vi "_nevstop_choosingDlg.vi"(8 "error in (no error)":errorcluster) -> (0 "error out":errorcluster, 1 "Cancelled?":bool=TRUE, 2 "QuckDrop":string, 3 "QDKS Info":T2[](array[typedef])=[{"VI Name"="Cluster AutoSizing", "VI Path"=path "C:/Program Files (x86)/National Instruments/LabVIEW 2014/resource/dialog/QuickDrop/plugins/QD_Cluster AutoSizing/Cluster AutoSizing.vi", "Default Shortcut"="U", "Assigned Shortcut"="u", "Description"="Using a float dialog to choose cluster auto-sizing type. Press `Shift` to set the contained cluster items recursively. \n\n- None\n- Size to Fit\n- Arrange Horizontally\n- Arrange Vertically\n\nDefault Shortcut - [U]"}, {"VI Name"="Align - Bottom Edges", "VI Path"=path "C:/Program Files (x86)/National Instruments/LabVIEW 2014/resource/dialog/QuickDrop/plugins/QD_Align&Distribute/Align - Bottom Edges.vi", "Default Shortcut"="v", "Assigned Shortcut"="v", "Description"="Align - Bottom Edges.vi\n"}, {"VI Name"="Align - Horizontal Centers", "VI Path"=path "C:/Program Files (x86)/National Instruments/LabVIEW 2014/resource/dialog/QuickDrop/plugins/QD_Align&Distribute/Align - Horizontal Centers.vi", "Default Shortcut"="v", "Assigned Shortcut"="", "Description"="Align - Horizontal Centers.vi"}, {"VI Name"="Align - Left Edges", "VI Path"=path "C:/Program Files (x86)/National Instruments/LabVIEW 2014/resource/dialog/QuickDrop/plugins/QD_Align&Distribute/Align - Left Edges.vi", "Default Shortcut"="v", "Assigned Shortcut"="5", "Description"="Align - Left Edges.vi"}, {"VI Name"="Align - Right Edges", "VI Path"=path "C:/Program Files (x86)/National Instruments/LabVIEW 2014/resource/dialog/QuickDrop/plugins/QD_Align&Distribute/Align - Right Edges.vi", "Default Shortcut"="v", "Assigned Shortcut"="", "Description"="Align - Right Edges.vi"}, {"VI Name"="Align - Top Edges", "VI Path"=path "C:/Program Files (x86)/National Instruments/LabVIEW 2014/resource/dialog/QuickDrop/plugins/QD_Align&Distribute/Align - Top Edges.vi", "Default Shortcut"="v", "Assigned Shortcut"="", "Description"="Align - Top Edges.vi"}, {"VI Name"="Align - Vertical Centers", "VI Path"=path "C:/Program Files (x86)/National Instruments/LabVIEW 2014/resource/dialog/QuickDrop/plugins/QD_Align&Distribute/Align - Vertical Centers.vi", "Default Shortcut"="v", "Assigned Shortcut"="", "Description"="Align - Vertical Centers.vi"}, {"VI Name"="Align and Distribute", "VI Path"=path "C:/Program Files (x86)/National Instruments/LabVIEW 2014/resource/dialog/QuickDrop/plugins/QD_Align&Distribute/Align and Distribute.vi", "Default Shortcut"="A", "Assigned Shortcut"="a", "Description"="Aligns selected items to the right, left, top or bottom or by horizontal or vertical centers by pressing r, l, t, b, h or v."}, {"VI Name"="Arrange VI Window", "VI Path"=path "C:/Program Files (x86)/National Instruments/LabVIEW 2014/resource/dialog/QuickDrop/plugins/QD_Arrange VI Window/Arrange VI Window.vi", "Default Shortcut"="F", "Assigned Shortcut"="f", "Description"="When used on the front panel:\n-Arranges controls and indicators to be consistent with the connector pane arrangement. \n-Resizes and moves the front panel to a consistent top left location on the primary monitor.\n\nWhen used on the block diagram:\n-Scrolls the block diagram to a reasonable location relative to the top-most and/or left-most diagram object.\n-Resizes and moves the block diagram to a consistent top left location on the primary monitor.\n\nDefault Shortcut - [F]"}, {"VI Name"="Build Array of References", "VI Path"=path "C:/Program Files (x86)/National Instruments/LabVIEW 2014/resource/dialog/QuickDrop/plugins/QD_Build Array of References/Build Array of References_NEVSTOP.vi", "Default Shortcut"="B", "Assigned Shortcut"="b", "Description"="### Build Array of Reference/Build Cluster of Reference\n\nCreate references with 'Build Array'/'buddle' together.\n\nDefault Shortcut - [B]"}, {"VI Name"="Build Cluster Of Reference", "VI Path"=path "C:/Program Files (x86)/National Instruments/LabVIEW 2014/resource/dialog/QuickDrop/plugins/QD_Build Cluster of References/Build Cluster Of Reference.vi", "Default Shortcut"="$", "Assigned Shortcut"="2", "Description"="Write a 1-2 sentence description of the functionality of your plugin here.  Replace the \"$\" below with the character you wish to assign as the default shortcut for this plugin.  Do not add any text after the 'Default Shortcut' line below.\n\nDefault Shortcut - [$]"}, {"VI Name"="Clone Control", "VI Path"=path "C:/Program Files (x86)/National Instruments/LabVIEW 2014/resource/dialog/QuickDrop/plugins/QD_Clone Control/Clone Control.vi", "Default Shortcut"="", "Assigned Shortcut"="", "Description"="Clones the selected Control(s) or Indicator(s) on the Front Panel but changes Controls to Indicators and vice versa.  In addition, if found on the Connector Pane, will attempt to place the newly created control on the opposite (left / right) side of the Connector Pane.\nNote: This script only supports the following patterns: 4x2x2x4, 5x3x3x5, 6x4x4x6, and 8x6x6x8.\n\nDefault Shortcut - [A]"}, {"VI Name"="Cluster AutoSizing - Arrange Horizontally", "VI Path"=path "C:/Program Files (x86)/National Instruments/LabVIEW 2014/resource/dialog/QuickDrop/plugins/QD_Cluster AutoSizing/Cluster AutoSizing - Arrange Horizontally.vi", "Default Shortcut"="v", "Assigned Shortcut"="", "Description"="Cluster AutoSizing - Arrange Horizontally.vi"}, {"VI Name"="Cluster AutoSizing - Arrange Veritcally", "VI Path"=path "C:/Program Files (x86)/National Instruments/LabVIEW 2014/resource/dialog/QuickDrop/plugins/QD_Cluster AutoSizing/Cluster AutoSizing - Arrange Veritcally.vi", "Default Shortcut"="v", "Assigned Shortcut"="", "Description"="Cluster AutoSizing - Arrange Veritcally.vi"}, {"VI Name"="Cluster AutoSizing - None", "VI Path"=path "C:/Program Files (x86)/National Instruments/LabVIEW 2014/resource/dialog/QuickDrop/plugins/QD_Cluster AutoSizing/Cluster AutoSizing - None.vi", "Default Shortcut"="v", "Assigned Shortcut"="", "Description"="Cluster AutoSizing - None.vi"}, {"VI Name"="Cluster AutoSizing - Size to Fit", "VI Path"=path "C:/Program Files (x86)/National Instruments/LabVIEW 2014/resource/dialog/QuickDrop/plugins/QD_Cluster AutoSizing/Cluster AutoSizing - Size to Fit.vi", "Default Shortcut"="v", "Assigned Shortcut"="", "Description"="Cluster AutoSizing - Size to Fit.vi"}, {"VI Name"="ColourUpStructures", "VI Path"=path "C:/Program Files (x86)/National Instruments/LabVIEW 2014/resource/dialog/QuickDrop/plugins/QD_ColourUpStructures/ColourUpStructures.vi", "Default Shortcut"="s", "Assigned Shortcut"="s", "Description"="Colour Up Structures."}, {"VI Name"="Copy Boolean Caption to BooleanText", "VI Path"=path "C:/Program Files (x86)/National Instruments/LabVIEW 2014/resource/dialog/QuickDrop/plugins/QD_Controls Operation/Copy Boolean Caption to BooleanText.vi", "Default Shortcut"="d", "Assigned Shortcut"="", "Description"="Copy selected boolean's caption to boolean text. If the booleans have no caption, label Text will be used instead."}, {"VI Name"="Create a Place VI Contents", "VI Path"=path "C:/Program Files (x86)/National Instruments/LabVIEW 2014/resource/dialog/QuickDrop/plugins/QD_Create a Place VI Contents/Create a Place VI Contents.vi", "Default Shortcut"="G", "Assigned Shortcut"="g", "Description"="(Note: The following shortcut was originally posted by Jarrod S. on the NI Forums here.  I decided to give his shortcut a more permanent home in the Quick Drop Enthusiasts group.)\n \nThis Quick Drop Keyboard Shortcut allows you to create a Place VI Contents VI (formerly called a \"Merge VI\") of your diagram selection and automatically create a user.lib palette entry for it, so that you can easily drop that selection of code in the future.  Follow these steps to use this shortcut:\n \nSave the attached VI in your <LabVIEW>\\resource\\dialog\\QuickDrop\\plugins folder.  No LabVIEW restart is required.\nSelect something on your diagram that you wish to make into a Place VI Contents VI.\nPress Ctrl-Space-Ctrl-Shift-G.\nSpecify a name for this Place VI Contents VI.\nCreate an icon\n \nNow you have a Place VI Contents VI that contains this diagram selection that you can use from your palettes (or Quick Drop).  Note that in step (3) above, if you had pressed Ctrl-Space-Ctrl-G instead, the palettes would not be refreshed automatically, and you would have to restart LabVIEW in order to use the new Place VI Contents VI.\n \nNote:  All Place VI Contents VIs that are created with this shortcut are stored in <LabVIEW Data>\\QuickDrop Templates.  The actual .mnu files that provide the palette entries are stored in <LabVIEW>\\user.lib\\QuickDrop Templates Palette.mnu.\n\n\nDefault Shortcut - [G]"}, {"VI Name"="Disable Controls", "VI Path"=path "C:/Program Files (x86)/National Instruments/LabVIEW 2014/resource/dialog/QuickDrop/plugins/QD_Controls Operation/Disable Controls.vi", "Default Shortcut"="l", "Assigned Shortcut"="l", "Description"="Disable Controls"}, {"VI Name"="Disable&Grayout Controls", "VI Path"=path "C:/Program Files (x86)/National Instruments/LabVIEW 2014/resource/dialog/QuickDrop/plugins/QD_Controls Operation/Disable&Grayout Controls.vi", "Default Shortcut"="l", "Assigned Shortcut"="", "Description"="Disable and grayout Controls"}, {"VI Name"="Distribute - Bottom Edges", "VI Path"=path "C:/Program Files (x86)/National Instruments/LabVIEW 2014/resource/dialog/QuickDrop/plugins/QD_Align&Distribute/Distribute - Bottom Edges.vi", "Default Shortcut"="v", "Assigned Shortcut"="", "Description"="Distribute - Bottom Edges.vi"}, {"VI Name"="Distribute - Horizontal Centers", "VI Path"=path "C:/Program Files (x86)/National Instruments/LabVIEW 2014/resource/dialog/QuickDrop/plugins/QD_Align&Distribute/Distribute - Horizontal Centers.vi", "Default Shortcut"="v", "Assigned Shortcut"="", "Description"="Distribute - Horizontal Centers.vi"}, {"VI Name"="Distribute - Horizontal Compress", "VI Path"=path "C:/Program Files (x86)/National Instruments/LabVIEW 2014/resource/dialog/QuickDrop/plugins/QD_Align&Distribute/Distribute - Horizontal Compress.vi", "Default Shortcut"="v", "Assigned Shortcut"="", "Description"="Distribute - Horizontal Compress.vi"}, {"VI Name"="Distribute - Horizontal Gap", "VI Path"=path "C:/Program Files (x86)/National Instruments/LabVIEW 2014/resource/dialog/QuickDrop/plugins/QD_Align&Distribute/Distribute - Horizontal Gap.vi", "Default Shortcut"="v", "Assigned Shortcut"="", "Description"="Distribute - Horizontal Gap.vi"}, {"VI Name"="Distribute - Left Edges", "VI Path"=path "C:/Program Files (x86)/National Instruments/LabVIEW 2014/resource/dialog/QuickDrop/plugins/QD_Align&Distribute/Distribute - Left Edges.vi", "Default Shortcut"="v", "Assigned Shortcut"="", "Description"="Distribute - Left Edges.vi"}, {"VI Name"="Distribute - Right Edges", "VI Path"=path "C:/Program Files (x86)/National Instruments/LabVIEW 2014/resource/dialog/QuickDrop/plugins/QD_Align&Distribute/Distribute - Right Edges.vi", "Default Shortcut"="v", "Assigned Shortcut"="", "Description"="Distribute - Right Edges.vi"}, {"VI Name"="Distribute - Top Edges", "VI Path"=path "C:/Program Files (x86)/National Instruments/LabVIEW 2014/resource/dialog/QuickDrop/plugins/QD_Align&Distribute/Distribute - Top Edges.vi", "Default Shortcut"="v", "Assigned Shortcut"="", "Description"="Distribute - Top Edges.vi"}, {"VI Name"="Distribute - Vertical Centers", "VI Path"=path "C:/Program Files (x86)/National Instruments/LabVIEW 2014/resource/dialog/QuickDrop/plugins/QD_Align&Distribute/Distribute - Vertical Centers.vi", "Default Shortcut"="v", "Assigned Shortcut"="", "Description"="Distribute - Vertical Centers.vi"}, {"VI Name"="Distribute - Vertical Compress", "VI Path"=path "C:/Program Files (x86)/National Instruments/LabVIEW 2014/resource/dialog/QuickDrop/plugins/QD_Align&Distribute/Distribute - Vertical Compress.vi", "Default Shortcut"="v", "Assigned Shortcut"="", "Description"="Distribute - Vertical Compress.vi"}, {"VI Name"="Distribute - Vertical Gap", "VI Path"=path "C:/Program Files (x86)/National Instruments/LabVIEW 2014/resource/dialog/QuickDrop/plugins/QD_Align&Distribute/Distribute - Vertical Gap.vi", "Default Shortcut"="v", "Assigned Shortcut"="", "Description"="Distribute - Vertical Gap.vi"}, {"VI Name"="EasyConvert", "VI Path"=path "C:/Program Files (x86)/National Instruments/LabVIEW 2014/resource/dialog/QuickDrop/plugins/EasyConvert.vi", "Default Shortcut"="e", "Assigned Shortcut"="7", "Description"="Typecast or convert a constant/control/VI/terminal into another. Will use other palette objects like U8 to String if the type string matches.\n\nHold shift while using Cntrl-E to always use the Typecase with constant instead of selecting based on the coded algorithm.\n\nDefault Shortcut - [e]"}, {"VI Name"="Enable Controls", "VI Path"=path "C:/Program Files (x86)/National Instruments/LabVIEW 2014/resource/dialog/QuickDrop/plugins/QD_Controls Operation/Enable Controls.vi", "Default Shortcut"="l", "Assigned Shortcut"="", "Description"="Enable Controls"}, {"VI Name"="Erease Data(Clear Data)", "VI Path"=path "C:/Program Files (x86)/National Instruments/LabVIEW 2014/resource/dialog/QuickDrop/plugins/QD_Erease Data/Erease Data(Clear Data).vi", "Default Shortcut"="E", "Assigned Shortcut"="e", "Description"="Clear control/Constant's data. Supported type:\n- Array\n- String\n- Listbox\n- MulticolumnListBox\n- Numeric\n- Table\n- Tree\n\nDefault Shortcut - [E]"}, {"VI Name"="Front Panel Clean-Up", "VI Path"=path "C:/Program Files (x86)/National Instruments/LabVIEW 2014/resource/dialog/QuickDrop/plugins/LMH-Toolbox/Front Panel Clean-Up.vi", "Default Shortcut"="$", "Assigned Shortcut"="4", "Description"="Write a 1-2 sentence description of the functionality of your plugin here.  Replace the \"$\" below with the character you wish to assign as the default shortcut for this plugin.  Do not add any text after the 'Default Shortcut' line below.\n\nDefault Shortcut - [$]"}, {"VI Name"="Hide Controls", "VI Path"=path "C:/Program Files (x86)/National Instruments/LabVIEW 2014/resource/dialog/QuickDrop/plugins/QD_Controls Operation/Hide Controls.vi", "Default Shortcut"="l", "Assigned Shortcut"="", "Description"="Hide Controls"}, {"VI Name"="Insert", "VI Path"=path "C:/Program Files (x86)/National Instruments/LabVIEW 2014/resource/dialog/QuickDrop/plugins/Insert.vi", "Default Shortcut"="I", "Assigned Shortcut"="i", "Description"="Inserts the object specified by name in the Quick Drop dialog box on the selected wire(s) on the diagram.  If [Shift] is also pressed, and multiple wires were selected, a single instance of the object is inserted on those wires.\n\nDefault Shortcut - [I]"}, {"VI Name"="JKI State Machine Helper", "VI Path"=path "C:/Program Files (x86)/National Instruments/LabVIEW 2014/resource/dialog/QuickDrop/plugins/JKI State Machine Helper__JKI_State_Machine_Helper.vi", "Default Shortcut"="j", "Assigned Shortcut"="j", "Description"="Launches JKI State Machine Helper.\n\nDefault Shortcut - [j]"}, {"VI Name"="Magic Delay Fairy", "VI Path"=path "C:/Program Files (x86)/National Instruments/LabVIEW 2014/resource/dialog/QuickDrop/plugins/Magic Delay Fairy/Magic Delay Fairy.vi", "Default Shortcut"="F", "Assigned Shortcut"="1", "Description"="Inserts a wait millisecond delay into selected error wires.\n\nDefault Shortcut - [F]"}, {"VI Name"="Move Labels", "VI Path"=path "C:/Program Files (x86)/National Instruments/LabVIEW 2014/resource/dialog/QuickDrop/plugins/Move Labels.vi", "Default Shortcut"="T", "Assigned Shortcut"="t", "Description"="Repositions the visible labels or captions of top-level front panel and block diagram objects to be consistent with the \"Default label position\" settings in Tools > Options. If [Shift] is also pressed, then all objects, including nested objects, are modified. If this shortcut is activated from the front panel, then controls and indicators are modified. If it is activated from the block diagram, then control and indicator terminals are modified. If panel or diagram objects were already selected when this shortcut is activated, only the selected objects that have visible labels or captions are modified.\n\nThe text justification of the modified labels and captions is also modified to be consistent with the new label or caption position.\n\nDefault Shortcut - [T]"}, {"VI Name"="NEVSTOP QD Shortcuts", "VI Path"=path "C:/Program Files (x86)/National Instruments/LabVIEW 2014/resource/dialog/QuickDrop/plugins/QD_NEVSTOP QD Shortcuts/NEVSTOP QD Shortcuts.vi", "Default Shortcut"="Q", "Assigned Shortcut"="q", "Description"="NEVSTOP Quickdrops. Using a choosing dialog for quick QD selection.\n\nDefault Shortcut - [Q]"}, {"VI Name"="Open Current VI Location in Explorer Window", "VI Path"=path "C:/Program Files (x86)/National Instruments/LabVIEW 2014/resource/dialog/QuickDrop/plugins/QD_Smart Open VI Location/Open Current VI Location.vi", "Default Shortcut"="w", "Assigned Shortcut"="", "Description"="Open Current VI Location in Explorer Window."}, {"VI Name"="Open Selected VI's Location in Explorer Window", "VI Path"=path "C:/Program Files (x86)/National Instruments/LabVIEW 2014/resource/dialog/QuickDrop/plugins/QD_Smart Open VI Location/Open Selected VI Location.vi", "Default Shortcut"="w", "Assigned Shortcut"="", "Description"="Open Selected VI's Location in Explorer Window."}, {"VI Name"="Refresh Palette", "VI Path"=path "C:/Program Files (x86)/National Instruments/LabVIEW 2014/resource/dialog/QuickDrop/plugins/QD_Create a Place VI Contents/Refresh Palette.vi", "Default Shortcut"="p", "Assigned Shortcut"="", "Description"="After some chane of Control/Function Pallette, you can manually update the pallette with this quickdrop.\n"}, {"VI Name"="Remove and Rewire", "VI Path"=path "C:/Program Files (x86)/National Instruments/LabVIEW 2014/resource/dialog/QuickDrop/plugins/Remove and Rewire.vi", "Default Shortcut"="R", "Assigned Shortcut"="r", "Description"="Removes the selected block diagram object(s) and any wires and constants connected to the selected object(s), and connects wires of identical data types that were wired to the inputs and outputs of the deleted object(s).\n\nDefault Shortcut - [R]"}, {"VI Name"="Replace", "VI Path"=path "C:/Program Files (x86)/National Instruments/LabVIEW 2014/resource/dialog/QuickDrop/plugins/Replace.vi", "Default Shortcut"="P", "Assigned Shortcut"="p", "Description"="Replaces the selected panel or diagram object(s) with the object specified by name in the Quick Drop dialog box.\n\nDefault Shortcut - [P]"}, {"VI Name"="Reset Origin", "VI Path"=path "C:/Program Files (x86)/National Instruments/LabVIEW 2014/resource/dialog/QuickDrop/plugins/QD_Controls Operation/Reset Origin.vi", "Default Shortcut"=")", "Assigned Shortcut"=")", "Description"="Reset the origin of the front panel or block diagram to (0,0).\n"}, {"VI Name"="Show Controls", "VI Path"=path "C:/Program Files (x86)/National Instruments/LabVIEW 2014/resource/dialog/QuickDrop/plugins/QD_Controls Operation/Show Controls.vi", "Default Shortcut"="l", "Assigned Shortcut"="", "Description"="Show Controls"}, {"VI Name"="Smart Open VI Locaiton in Explorer Window", "VI Path"=path "C:/Program Files (x86)/National Instruments/LabVIEW 2014/resource/dialog/QuickDrop/plugins/QD_Smart Open VI Location/Smart Open VI Locaiton.vi", "Default Shortcut"="O", "Assigned Shortcut"="o", "Description"="When triggered on Front Panel:\nOpen Current VI's Location in Explorer Window.\n\nWhen triggered on Block Diagram:\nNo SubVI is selected: Open Current VI's Location in Explorer Window.\nSubVIs are selected: Open Selected VI's Location in Explorer Window.\n\nDefault Shortcut - [O]"}, {"VI Name"="State Machine from Enum", "VI Path"=path "C:/Program Files (x86)/National Instruments/LabVIEW 2014/resource/dialog/QuickDrop/plugins/QD_State Machine From Enum/_old version/State Machine from Enum (2010).vi", "Default Shortcut"="s", "Assigned Shortcut"="", "Description"="Creates a state machine from a selected enum."}, {"VI Name"="Toggle Digital Increment Decrement Visible ( Swithc Show Or Hide )", "VI Path"=path "C:/Program Files (x86)/National Instruments/LabVIEW 2014/resource/dialog/QuickDrop/plugins/QD_Controls Operation/Toggle Digital Increment Decrement Visible ( Swithc Show Or Hide ).vi", "Default Shortcut"="v", "Assigned Shortcut"="", "Description"="Toggle Digital Increment Decrement Visible ( Swithc Show Or Hide ).vi"}, {"VI Name"="VI Server Rename", "VI Path"=path "C:/Program Files (x86)/National Instruments/LabVIEW 2014/resource/dialog/QuickDrop/plugins/VI Server Rename.vi", "Default Shortcut"="B", "Assigned Shortcut"="0", "Description"="Changes the VI Server class of the selected property node(s), invoke node(s), and/or Class Specifier Constants, to the class typed in the Quick Drop window.  If [Shift] is also pressed, changes the property/method of the selected property node(s)/invoke node(s), respectively, to the property/method name typed in the Quick Drop window.\n\nDefault Shortcut - [B]"}, {"VI Name"="While Loop Subdiagram Label", "VI Path"=path "C:/Program Files (x86)/National Instruments/LabVIEW 2014/resource/dialog/QuickDrop/plugins/QD_While Loop Subdiagram Label/While Loop Subdiagram Label.vi", "Default Shortcut"="r", "Assigned Shortcut"="", "Description"="Takes the text in the Quick Drop box and applies it as a subdiagram label to a While Loop, and formats the subdiagram label to have white, bold text, with the while loop's gray background color."}, {"VI Name"="Wire All Terminals", "VI Path"=path "C:/Program Files (x86)/National Instruments/LabVIEW 2014/resource/dialog/QuickDrop/plugins/Wire All Terminals.vi", "Default Shortcut"="D", "Assigned Shortcut"="d", "Description"="Creates controls and indicators for all unwired inputs and outputs of the selected block diagram object(s).  If 'shift' is also pressed, creates constants for all unwired inputs of the selected block diagram object(s).\n\nDefault Shortcut - [D]"}, {"VI Name"="Wire Multiple Objects Together", "VI Path"=path "C:/Program Files (x86)/National Instruments/LabVIEW 2014/resource/dialog/QuickDrop/plugins/Wire Multiple Objects Together.vi", "Default Shortcut"="W", "Assigned Shortcut"="w", "Description"="Connects compatible terminals between multiple selected diagram objects. This shortcut will wire compatible data types between the objects in a left-to-right fashion. If [Shift] is also pressed, LabVIEW will perform a diagram cleanup of the selected objects after wiring them together.\n\nDefault Shortcut - [W]"}], 4 "Shift Pressed":bool)   [LabVIEW 2017, in "NEVSTOP QD Shortcuts.lvlib"]
uses:
  NEVSTOP QD Shortcuts.lvlib
  <resource>/dialog/QuickDrop/QuickDrop QDKS Info.ctl
  <vilib>/event_ctls.llb/eventvkey.ctl
panel:
  out "Path":path
  in  "[Trigger]Decorate List":bool=TRUE
  out "Variant":variant=variant("Align - Horizontal Centers"=variant(i32 2), "Align - Left Edges"=variant(i32 1), "Align and Distribute"=variant(i32 1), "Arrange VI Window"=variant(i32 1), "Build Array of References"=variant(i32 2), "Build Cluster Of Reference"=variant(i32 3), "Clone Control"=variant(i32 2), "Cluster AutoSizing"=variant(i32 4), "Cluster AutoSizing - None"=variant(i32 1), "Create a Place VI Contents"=variant(i32 1), "Distribute - Right Edges"=variant(i32 1), "Distribute - Vertical Compress"=variant(i32 1), "EasyConvert"=variant(i32 2), "Format Numeric"=variant(i32 1), "Front Panel Clean-Up"=variant(i32 4), "Move Labels"=variant(i32 1), "NEVSTOP QD Shortcuts"=variant(i32 1), "Show Controls"=variant(i32 1))
  in  "[Trigger]Update QSDK Info":bool=TRUE
  in  "[Trigger]Refresh Btns":bool=TRUE
  out "VKey":T1=enum."Escape"
  out "Info":string
  in  "FilterStr":string
  in  "Debug":bool
  out "Shift TEMP":bool
  in  "Shift":bool
  in  "M":bool caption="0"
  in  "N":bool caption="0"
  in  "L":bool caption="0"
  in  "K":bool caption="0"
  in  "J":bool caption="0"
  in  "H":bool caption="0"
  in  "P":bool caption="0"
  in  "O":bool caption="0"
  in  "I":bool caption="0"
  in  "U":bool caption="4"
  in  "Y":bool caption="0"
  in  "B":bool caption="2"
  in  "V":bool caption="0"
  in  "C":bool caption="0"
  in  "X":bool caption="0"
  in  "Z":bool caption="0"
  in  "G":bool caption="1"
  in  "F":bool caption="1"
  in  "D":bool caption="0"
  in  "S":bool caption="0"
  in  "A":bool caption="1"
  in  "T":bool caption="1"
  in  "R":bool caption="0"
  in  "E":bool caption="0"
  in  "W":bool caption="0"
  in  "Q":bool caption="1"
  in  "0":bool
  in  "9":bool caption="0"
  in  "8":bool caption="0"
  in  "7":bool caption="2"
  in  "6":bool caption="0"
  in  "5":bool caption="1"
  in  "4":bool
  in  "3":bool caption="0"
  in  "2":bool caption="3"
  in  "1":bool caption="0"
  in  "Listbox":i32(listbox)=-1
  out "Key Temp":string
  out "Char":i16
  # "Drag To Button, Change Assigned Shortcut, Drag to Shift, Clear Arrsigned Shortcut."
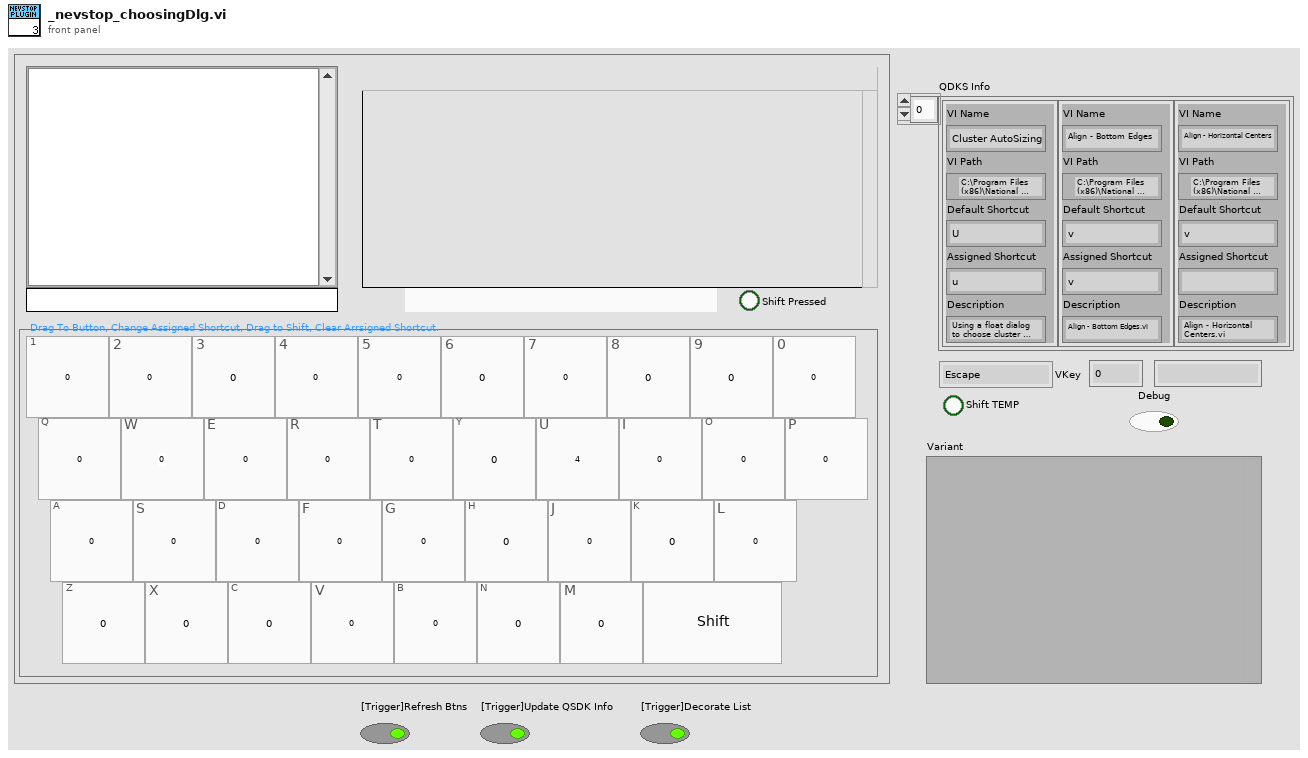
[diagram p1: front panel]
types:
  T1 = typedef "eventvkey.ctl" = enum16{"ASCII", "Enter", "Return", "Shift", "Ctrl", "Alt", "Cmd", "Opt", "Caps", "NumLock", "Clear", "Break", "Up", "Down", "Left", "Right", "Insert", "Delete", "Home", "End", "PageUp", "PageDown", "Escape", "Help", "Pause", "ScrollLock", "F1", "F2", "F3", "F4", "F5", "F6", "F7", "F8", "F9", "F10", "F11", "F12", "F13", "F14", "F15", "F16", "F17", "F18", "F19", "F20", "F21", "F22", "F23", "F24", "Play", "VolumeUp", "VolumeDown", "Mute", "Two Byte Char"}
  T2 = typedef "QuickDrop QDKS Info.ctl" = cluster{"VI Name":string, "VI Path":path, "Default Shortcut":string, "Assigned Shortcut":string, "Description":string}
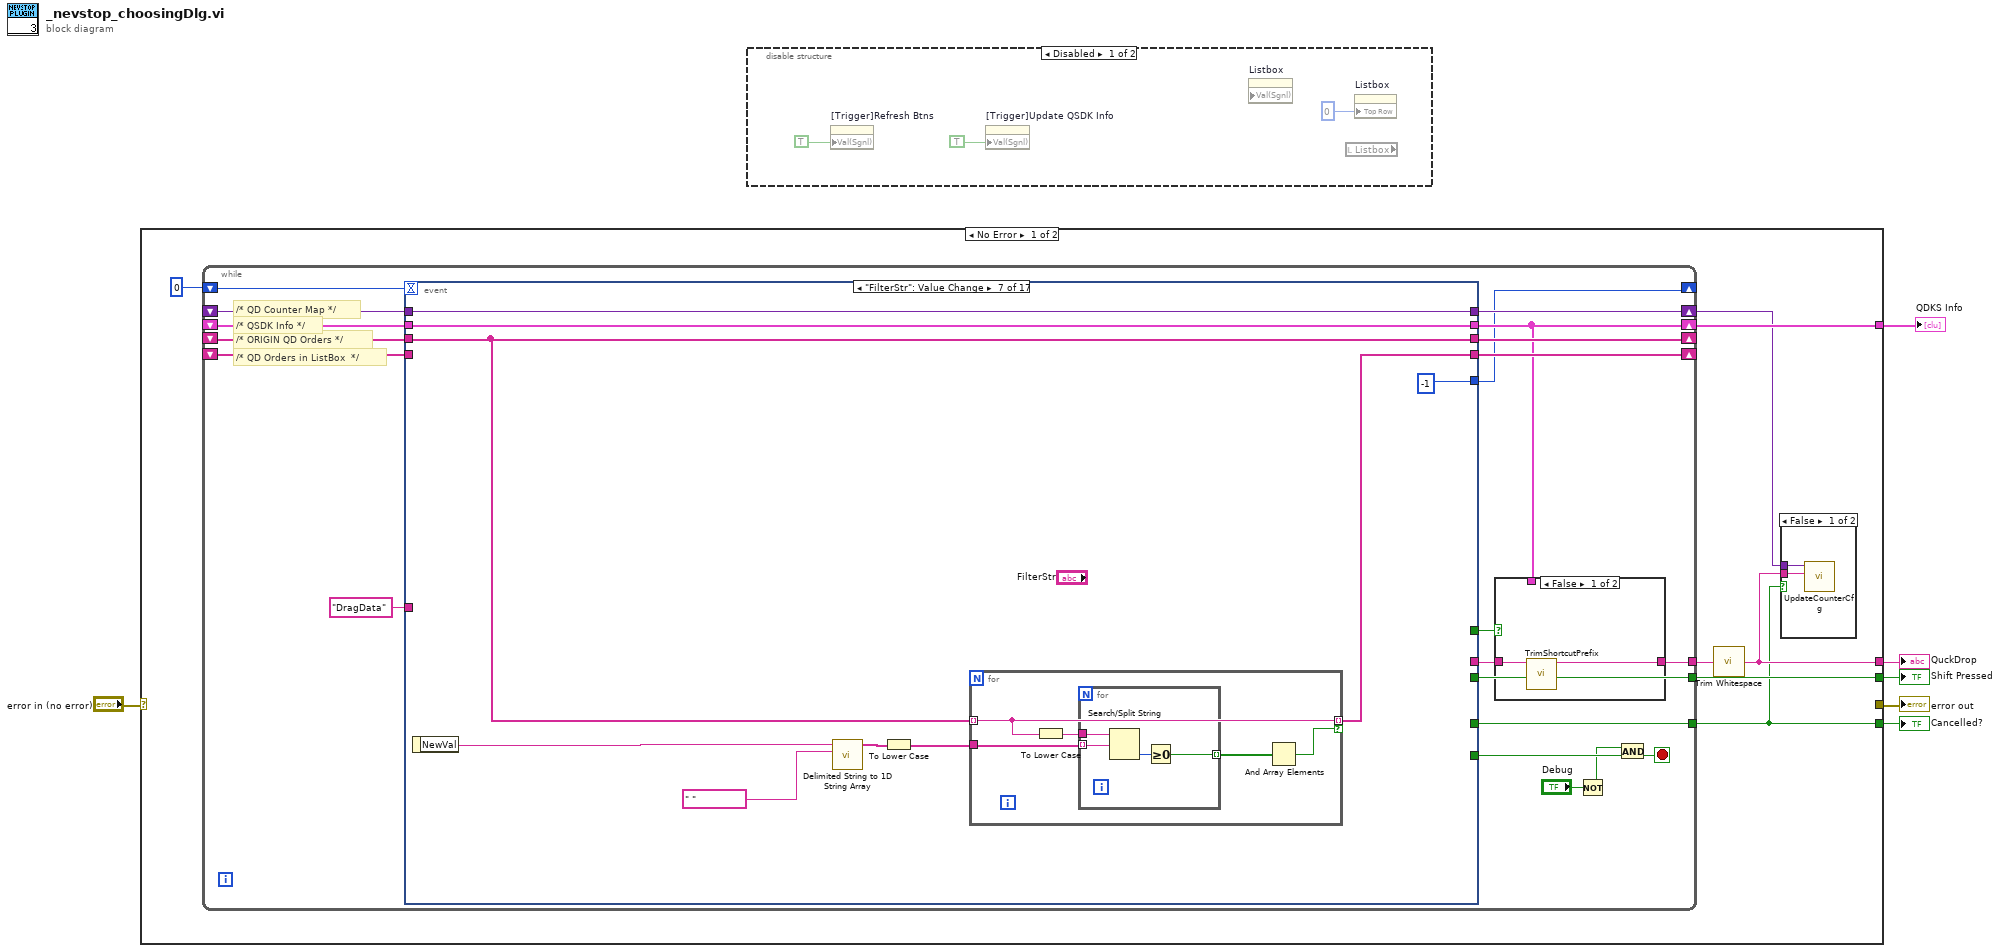
[diagram p0: block diagram]
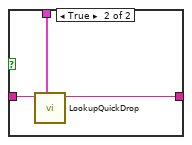
[diagram p4: hidden frame]
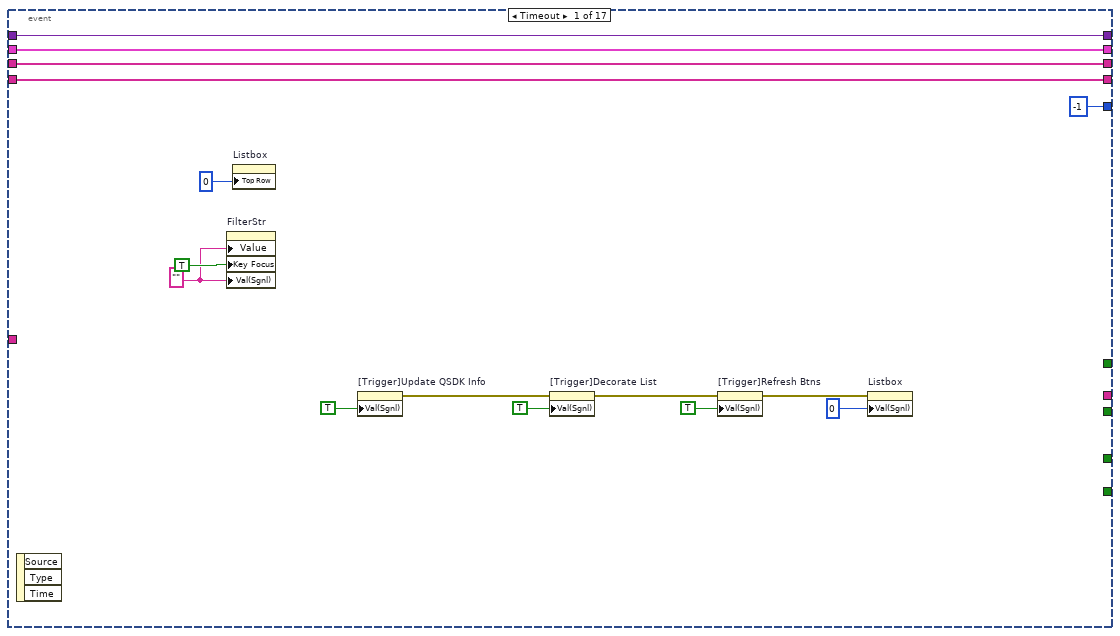
[diagram p5: hidden frame]
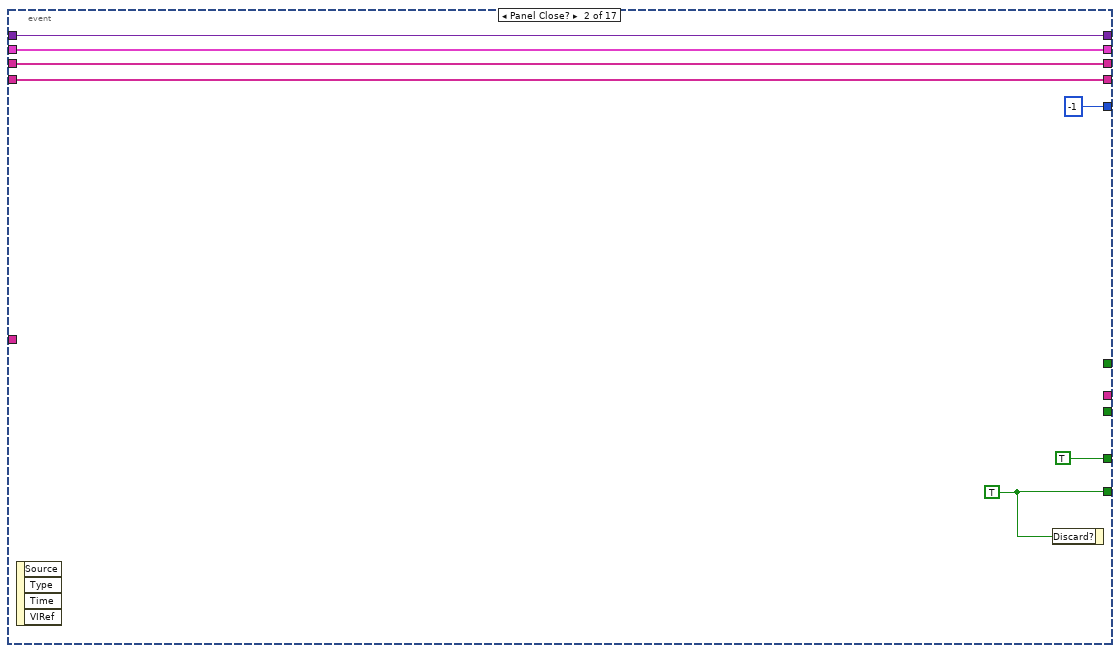
[diagram p6: hidden frame]
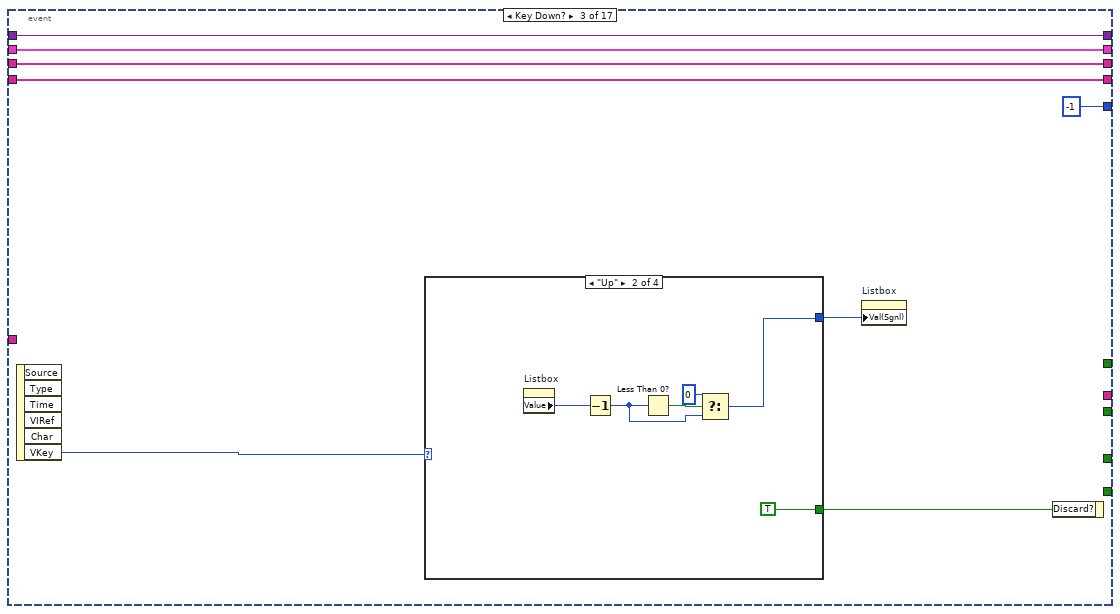
[diagram p7: hidden frame]
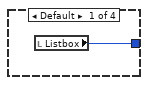
[diagram p8: hidden frame]
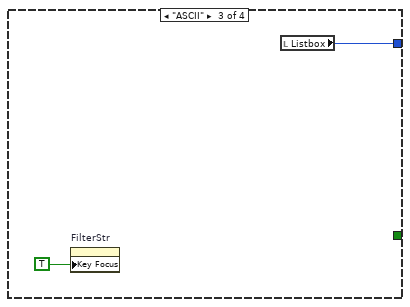
[diagram p9: hidden frame]
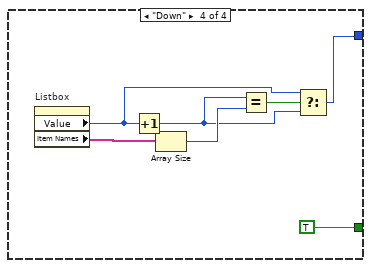
[diagram p10: hidden frame]
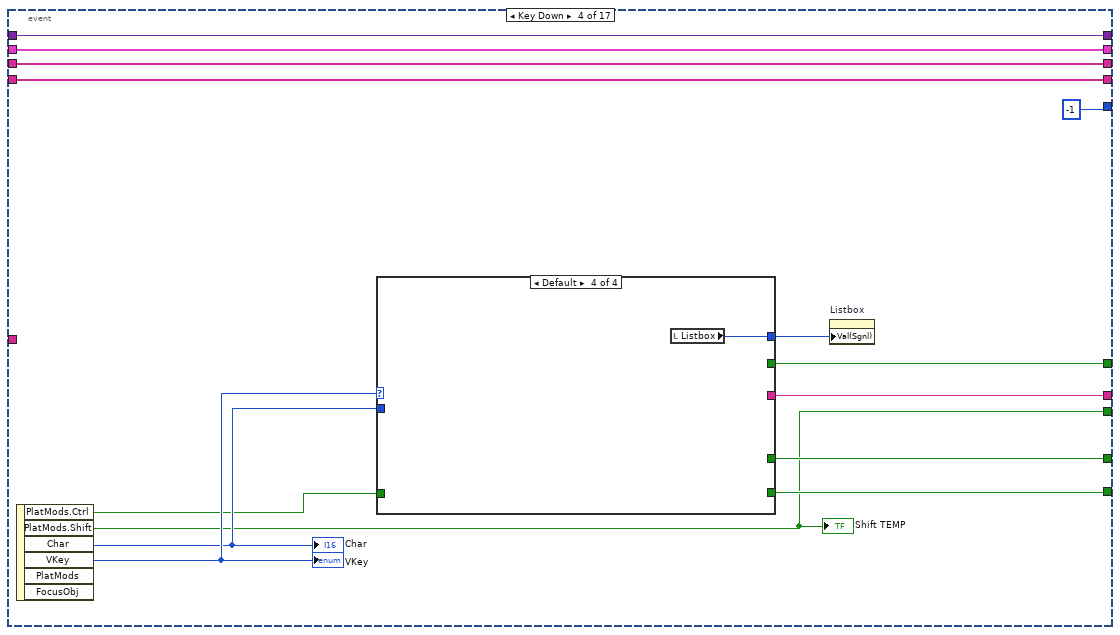
[diagram p11: hidden frame]
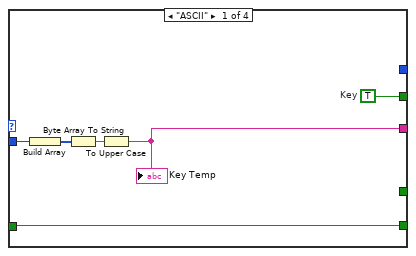
[diagram p12: hidden frame]
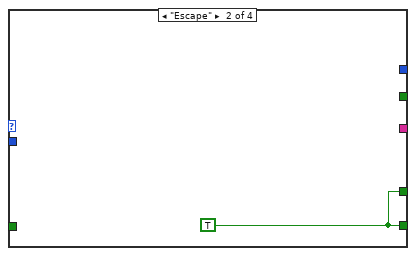
[diagram p13: hidden frame]
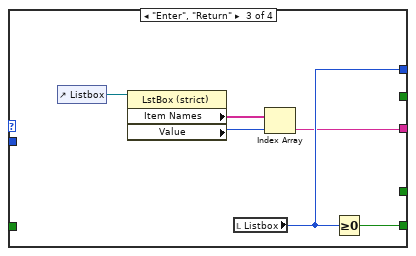
[diagram p14: hidden frame]
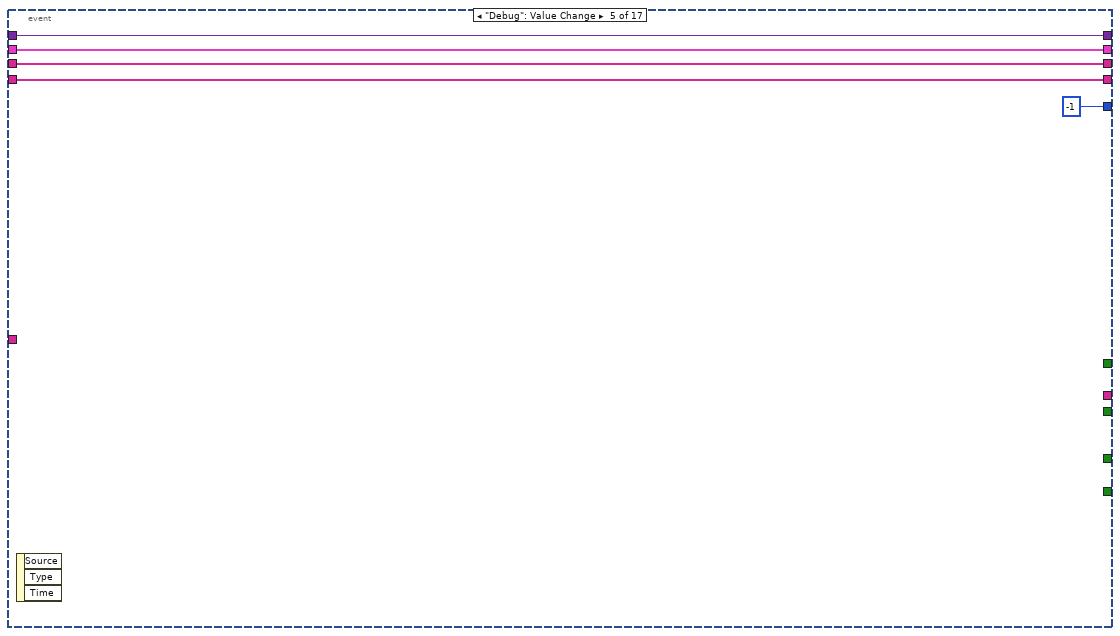
[diagram p15: hidden frame]
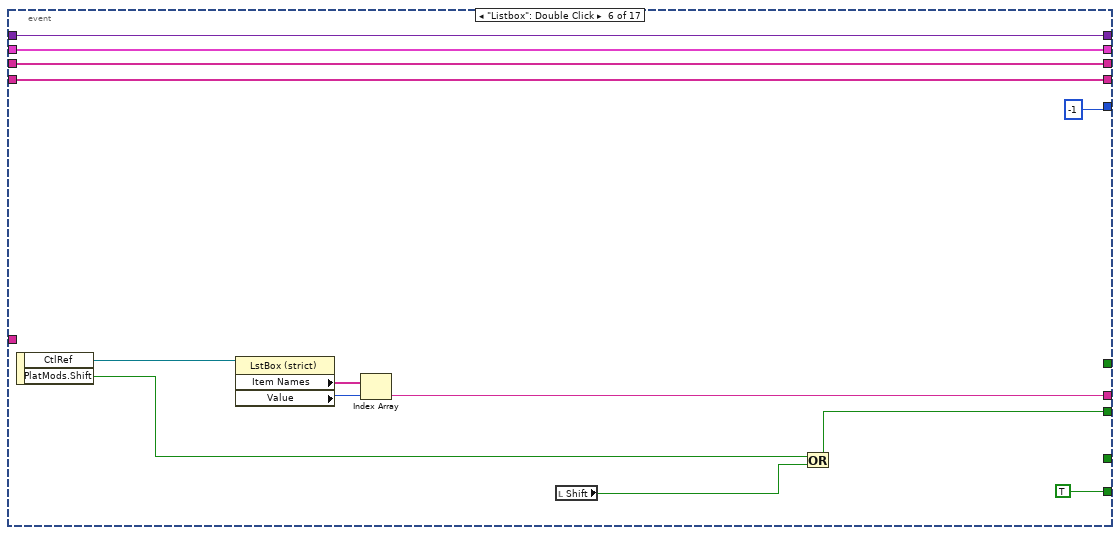
[diagram p16: hidden frame]
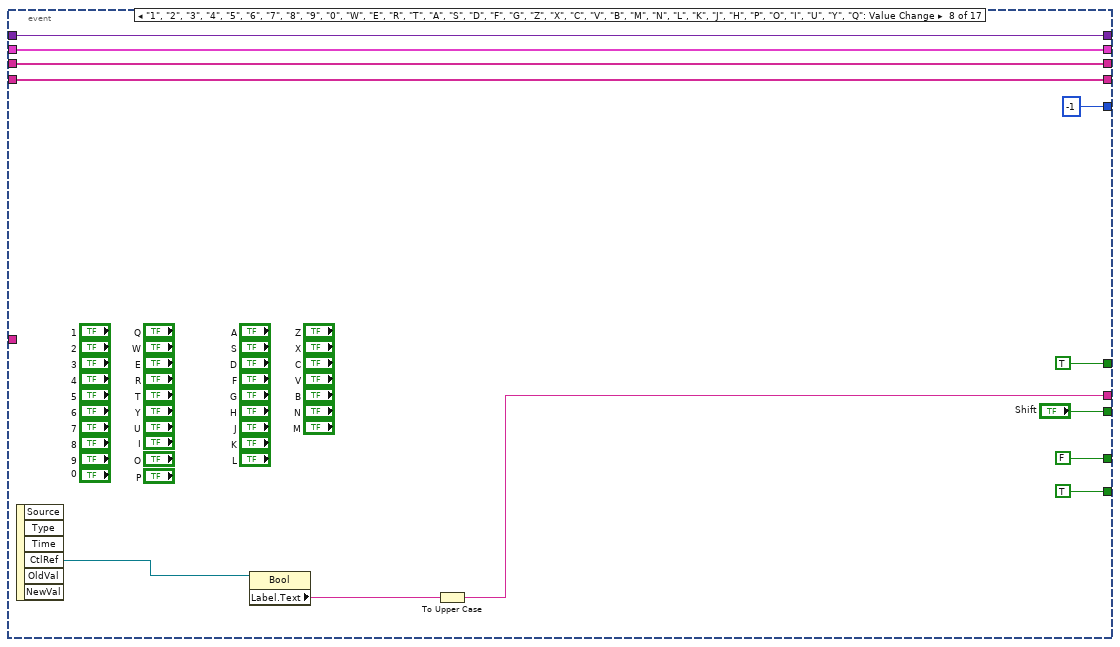
[diagram p17: hidden frame]
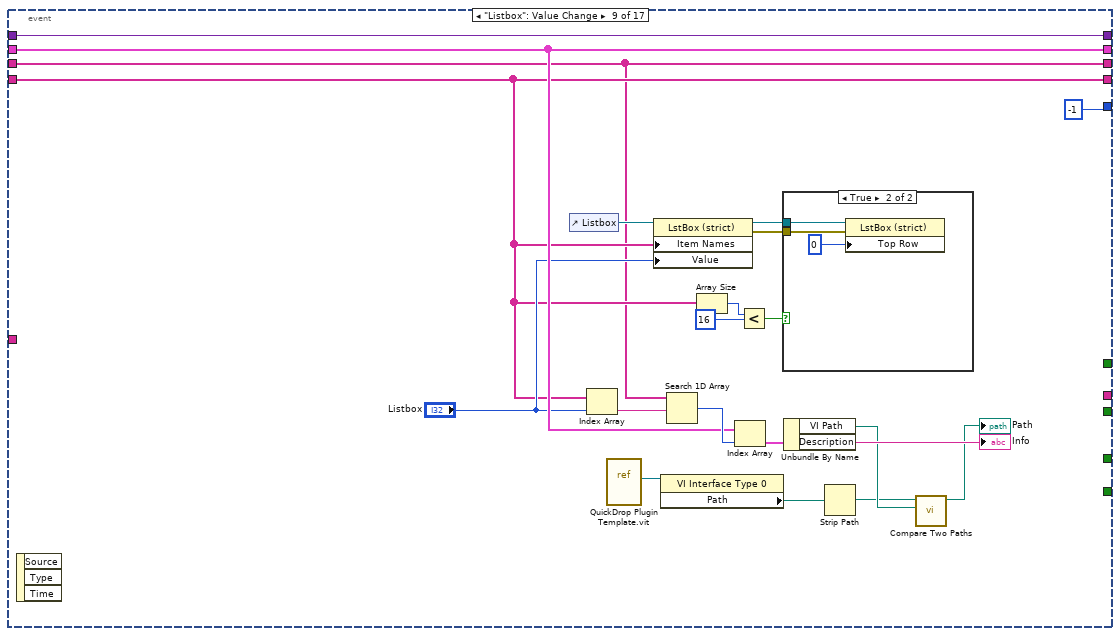
[diagram p18: hidden frame]
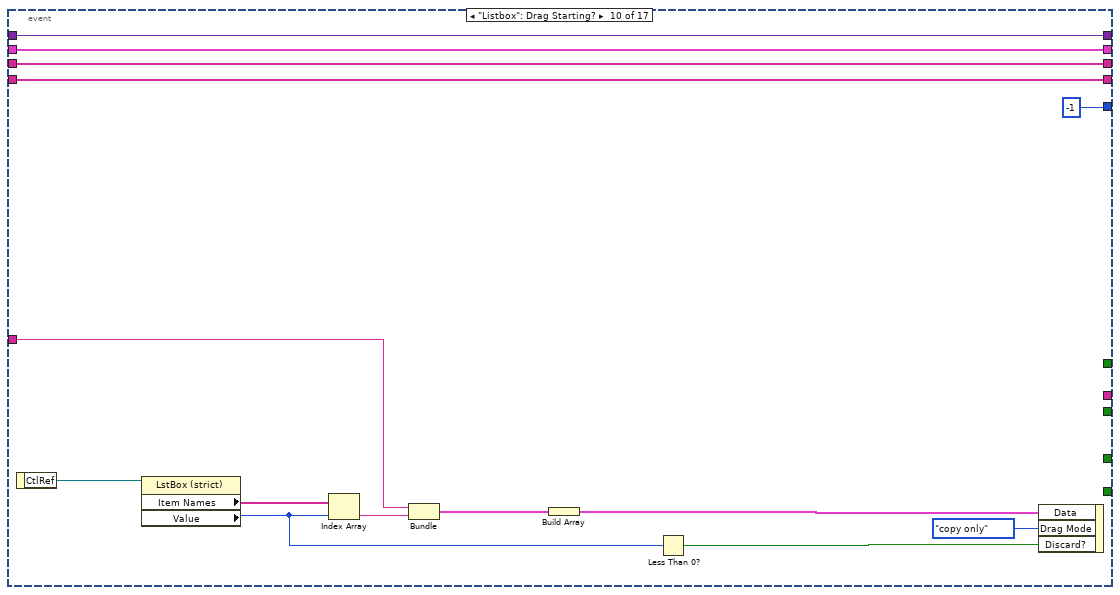
[diagram p20: hidden frame]
diagram:
  n1 = case shown="No Error" "error in (no error)" {
    selector: "error in (no error)" -> [_ w360]
    tunnel: [w7 TRUE] -> w6
    tunnel: [_ w360] -> w4
    tunnel: [w9 _] -> w3
    tunnel: [w11 _] -> w2
    tunnel: [w10 _] -> w1
    frame No Error {
      n2 = while {
        shift-right: [w16] -> _
        shift-left: 0 -> [w34]
        tunnel: [w33] -> w7
        tunnel: [w27] -> w12
        tunnel: [w32] -> w11
        shift-right: [w22] -> _
        shift-left: _ -> [w25]
        shift-right: [w17] -> w10
        shift-left: _ -> [w24]
        shift-right: [w20] -> _
        shift-left: _ -> [w23]
        shift-right: [w19] -> w8
        shift-left: _ -> [w18]
        stop <- w31 stop-if-true
        # "/* QD Orders in ListBox  */"
        # "/* ORIGIN QD Orders */"
        # "/* QD Counter Map */"
        # "/* QSDK Info */"
        n3 = event shown="[6] \"FilterStr\": Value Change" {
          selector: _ -> [_ _ _ _ _ _ _ _ _ _ _ _ _ _ _ _ _]
          dyn-events: _ -> [_ _ _ _ _ _ _ _ _ _ _ _ _ _ _ _ _]
          timeout: w34 -> [_ _ _ _ _ _ _ _ _ _ _ _ _ _ _ _ _]
          tunnel: [_ w62 _ w97 _ TRUE ("Discard?") _ TRUE ("Discard?") _ _ _ _ _ _ _ _ _] -> w35
          tunnel: [_ TRUE _ w96 _ _ _ FALSE _ _ _ _ _ _ _ _ _] -> w33
          tunnel: [_ _ _ w98 _ w129 _ w158 _ _ _ _ _ _ _ _ _] -> w26
          tunnel: [_ _ _ w95 _ w127 _ "Shift" _ _ _ _ _ _ _ _ _] -> w32
          tunnel: [_ _ _ w92 _ _ _ TRUE ("Key") _ _ _ _ _ _ _ _ _] -> w28
          tunnel: w24 -> [w51 w59 w67 w91 w118 w123 w137 w154 w172 w190 w204 w223 w232 w254 _ w333 w338]
          tunnel: [w54 w60 w70 w94 w119 w125 w140 w155 w170 w200 w211 w228 w240 w271 w287 w334 w339] -> w22
          tunnel: w25 -> [w54 w60 w70 w94 w119 w125 _ w155 w170 w200 w211 w228 w240 w271 _ w334 _]
          tunnel: w23 -> [w50 w58 w66 w90 w117 w122 w141 w153 w169 w189 w203 w222 w231 w253 _ w332 _]
          tunnel: "DragData" -> [_ _ _ _ _ _ _ _ _ w193 w209 w226 w238 _ _ _ _]
          tunnel: [w51 w59 w67 w91 w118 w123 w137 w154 w172 w190 w204 w223 w232 w254 w288 w333 w338] -> w17
          tunnel: [w50 w58 w66 w90 w117 w122 w141 w153 w169 w189 w203 w222 w231 w253 w287 w332 w339] -> w20
          tunnel: [w48 w57 w65 w89 w116 w121 w136 w152 w183 w188 w202 w221 w230 w252 w286 w331 w335] -> w19
          tunnel: w18 -> [w48 w57 w65 w89 w116 w121 w136 w152 w183 w188 w202 w221 w230 w252 _ w331 w336]
          tunnel: [-1 -1 -1 -1 -1 -1 -1 -1 -1 -1 0 -1 0 -1 -1 -1 -1] -> w16
          event Timeout {
            w53 = "" ("Value (Signaling)")
            n4 = event-data() -> ()  [unwired: 1 in, 3 out]
            n5 = property on="FilterStr" class="Str"("Value"=w53, "Key Focus"=TRUE, "Val(Sgnl)"=w53) -> ()  [unwired: 2 in, 2 out]
            n6 = property on="Listbox" class="LstBox (strict)"("Top Row"=0) -> ()  [unwired: 2 in, 2 out]
            n7 = property on="[Trigger]Update QSDK Info" class="Bool (strict)"("Val(Sgnl)"=TRUE ("Value (Signaling)")) -> (error out=w44:errorcluster)  [unwired: 2 in, 1 out]
            n8 = property on="[Trigger]Decorate List" class="Bool (strict)"(error in=w44, "Val(Sgnl)"=TRUE ("Value (Signaling)")) -> (error out=w43:errorcluster)  [unwired: 1 in, 1 out]
            n9 = property on="[Trigger]Refresh Btns" class="Bool (strict)"(error in=w43, "Val(Sgnl)"=TRUE ("Value (Signaling)")) -> (error out=w47:errorcluster)  [unwired: 1 in, 1 out]
            n10 = property on="Listbox" class="LstBox (strict)"(error in=w47, "Val(Sgnl)"=0) -> ()  [unwired: 1 in, 2 out]
          }
          event Panel Close? {
            w62 = TRUE ("Discard?")
            n11 = event-data() -> ()  [unwired: 1 in, 4 out]
            n12 = event-data("Discard?"=w62) -> ()  [unwired: 1 in, 1 out]
          }
          event Key Down? {
            n13 = event-data() -> ("VKey"=w69:T1)  [unwired: 1 in, 5 out]
            n14 = case shown="\"Up\"" w69 {
              tunnel: [_ TRUE _ TRUE] -> w68
              tunnel: [w71 w72 w79 w80] -> w64
              frame Default {
                n15 = local read "Listbox"() -> (w71:i32)
              }
              frame "Up" {
                n16 = property on="Listbox" class="LstBox (strict)"() -> ("Value"=w76:i32)  [unwired: 2 in, 2 out]
                n17 = Decrement(x=w76) -> (x-1=w73:i32)
                n18 = Less Than 0?(x=w73) -> (x < 0?=w75:bool)
                n19 = Select(t=0, s=w75, f=w73) -> (s? t:f=w72:i32)
              }
              frame "ASCII" {
                n20 = property on="FilterStr" class="Str"("Key Focus"=TRUE) -> ()  [unwired: 2 in, 2 out]
                n21 = local read "Listbox"() -> (w79:i32)
              }
              frame "Down" {
                n22 = property on="Listbox" class="LstBox (strict)"() -> ("Value"=w81:i32, "Item Names"=w85:string[])  [unwired: 2 in, 2 out]
                n23 = Increment(x=w81) -> (x+1=w82:i32)
                n24 = Array Size(array=w85) -> (size(s)=w84:i32)
                n25 = Equal?(x=w82, y=w84) -> (x = y?=w83:bool)
                n26 = Select(t=w81, s=w83, f=w82) -> (s? t:f=w80:i32)
              }
            }
            n27 = property on="Listbox" class="LstBox (strict)"("Val(Sgnl)"=w64) -> ()  [unwired: 2 in, 2 out]
            n28 = event-data("Discard?"=w68) -> ()  [unwired: 1 in, 1 out]
          }
          event Key Down {
            n29 = event-data() -> ("PlatMods.Ctrl"=w93:bool, "PlatMods.Shift"=w95:bool, "Char"=w99:i16, "VKey"=w100:T1)  [unwired: 1 in, 2 out]
            "Char" <- w99
            "Shift TEMP" <- w95
            "VKey" <- w100
            n30 = case shown="Default" w100 {
              tunnel: w99 -> [w106 _ _ _]
              tunnel: [w103 _ w108 _] -> w98
              tunnel: [w102 w107 w113 _] -> w97
              tunnel: [_ w107 _ _] -> w96
              tunnel: w93 -> [w102 _ _ _]
              tunnel: [w101 _ _ _] -> w92
              tunnel: [_ _ w112 w114] -> w88
              frame "ASCII" {
                w101 = TRUE  # Key
                n31 = Build Array(w106) -> (w105:i16[])
                n32 = Byte Array To String(unsigned byte array=w105) -> (string=w104:string)
                n33 = To Upper Case(1:w104) -> (0:w103:string)
                "Key Temp" <- w103
              }
              frame "Escape" {
                w107 = TRUE
              }
              frame "Enter", "Return" {
                n34 = control-ref of="Listbox"() -> (w111:refnum<vi>)
                n35 = property on="Property Node" class="LstBox (strict)"(reference=w111) -> ("Item Names"=w110:string[], "Value"=w109:i32)  [unwired: 1 in, 2 out]
                n36 = local read "Listbox"() -> (w112:i32)
                n37 = Index Array(array=w110, index=w109) -> (element=w108:string)
                n38 = Greater Or Equal To 0?(x=w112) -> (x >= 0?=w113:bool)
              }
              frame Default {
                n39 = local read "Listbox"() -> (w114:i32)
              }
            }
            n40 = property on="Listbox" class="LstBox (strict)"("Val(Sgnl)"=w88) -> ()  [unwired: 2 in, 2 out]
          }
          event "Debug": Value Change {
            n41 = event-data() -> ()  [unwired: 1 in, 3 out]
          }
          event "Listbox": Double Click {
            n42 = event-data() -> ("CtlRef"=w131:refnum<vi>, "PlatMods.Shift"=w126:bool)  [unwired: 1 in]
            n43 = property class="LstBox (strict)"(reference=w131) -> ("Item Names"=w130:string[], "Value"=w124:i32)  [unwired: 1 in, 2 out]
            n44 = Index Array(array=w130, index=w124) -> (element=w129:string)
            n45 = local read "Shift"() -> (w128:bool)
            n46 = Or(x=w126, y=w128) -> (x .or. y?=w127:bool)
          }
          event "FilterStr": Value Change {
            n47 = event-data() -> ("NewVal"=w134:string)  [unwired: 1 in]
            n48 = call "Delimited String to 1D String Array.vi"("delimiter"=" " ("delimiter (Tab)"), "delimited string"=w134) -> ("string array"=w139:string[])  [unwired: 9 in]
            n49 = To Lower Case(string=w139) -> (all lower case string=w138:string[])
            n50 = for {
              tunnel: w141 -> [w145] mode=indexing
              tunnel: w138 -> [w146]
              tunnel: [w145] -> w140 mode=indexing if=w142
              n51 = To Lower Case(string=w145) -> (all lower case string=w143:string)
              n52 = for {
                tunnel: [w149] -> w144 mode=indexing
                tunnel: w143 -> [w148]
                tunnel: w146 -> [w147] mode=indexing
                n53 = Search/Split String(string=w148, search string/char (-)=w147) -> (offset of match=w150:i32)  [unwired: 1 in, 2 out]
                n54 = Greater Or Equal To 0?(x=w150) -> (x >= 0?=w149:bool)
              }
              n55 = And Array Elements(Boolean array=w144) -> (logical AND=w142:bool)
            }
          }
          event "1", "2", "3", "4", "5", "6", "7", "8", "9", "0", "W", "E", "R", "T", "A", "S", "D", "F", "G", "Z", "X", "C", "V", "B", "M", "N", "L", "K", "J", "H", "P", "O", "I", "U", "Y", "Q": Value Change {
            n56 = event-data() -> ("CtlRef"=w162:refnum<vi>)  [unwired: 1 in, 5 out]
            n57 = property class="Bool"(reference=w162) -> ("Label.Text"=w161:string)  [unwired: 1 in, 2 out]
            n58 = To Upper Case(1:w161) -> (0:w158:string)
          }
          event "Listbox": Value Change {
            n59 = event-data() -> ()  [unwired: 1 in, 3 out]
            n60 = control-ref of="Listbox"() -> (w179:refnum<vi>)
            n61 = Index Array(array=w170, index="Listbox") -> (element=w176:string)
            n62 = vi-ref <resource>:"QuickDrop Plugin Template.vit"() -> (w167:refnum<vi>)
            n63 = property on="Property Node" class="LstBox (strict)"(reference=w179, "Item Names"=w170, "Value"="Listbox") -> (reference out=w178:refnum<vi>, error out=w177:errorcluster)  [unwired: 1 in]
            n64 = property class="VI Interface Type 0"(reference=w167) -> ("Path"=w166:path)  [unwired: 1 in, 2 out]
            n65 = Search 1D Array(1D array=w169, element=w176) -> (index of element=w173:i32)  [unwired: 1 in]
            n66 = Array Size(array=w170) -> (size(s)=w180:i32)
            n67 = Index Array(array=w172, index=w173) -> (element=w174:T2)
            n68 = Less?(x=w180, y=16) -> (x < y?=w182:bool)
            n69 = case shown="True" w182 {
              tunnel: w177 -> [_ w186]
              tunnel: w178 -> [_ w185]
              frame False {
              }
              frame True {
                n70 = property on="Property Node" class="LstBox (strict)"(reference=w185, error in=w186, "Top Row"=0) -> ()  [unwired: 2 out]
              }
            }
            n71 = Unbundle By Name(w174) -> ("VI Path"=w165:path, "Description"=→"Info":string)
            n72 = Strip Path(path=w166) -> (stripped path=w164:path)  [unwired: 1 out]
            n73 = call <vilib>:"Compare Two Paths.vi"("Path 2"=w165, "Path 1"=w164) -> ("Relative Path from 1 to 2"=→"Path":path)  [unwired: 6 in, 3 out]
          }
          event "Listbox": Drag Starting? {
            n74 = event-data() -> ("CtlRef"=w198:refnum<vi>)  [unwired: 1 in]
            n75 = property class="LstBox (strict)"(reference=w198) -> ("Item Names"=w196:string[], "Value"=w195:i32)  [unwired: 1 in, 2 out]
            n76 = Index Array(array=w196, index=w195) -> (element=w194:string)
            n77 = Bundle(w193, w194) -> (w192:cluster{string, string})  [unwired: 1 in]
            n78 = Build Array(w192) -> (w191:cluster{string, string}[])
            n79 = Less Than 0?(x=w195) -> (x < 0?=w197:bool)
            n80 = event-data("Data"=w191, "Drag Mode"=enum32{"copy or move", "copy only", "move only"}."copy only", "Discard?"=w197) -> ()  [unwired: 1 in, 1 out]
          }
          event "Shift": Drop {
            # "/* Force Refresh */"
            n81 = event-data() -> ("CtlRef"=w207:refnum<vi>, "Available Data Names"=w210:string[])  [unwired: 1 in, 4 out]
            n82 = Search 1D Array(1D array=w210, element=w209) -> (index of element=w208:i32)  [unwired: 1 in]
            n83 = case shown="0.." w208 {
              tunnel: w209 -> [_ w219]
              tunnel: [_ TRUE] -> w206
              tunnel: w207 -> [_ _]
              tunnel: [_ w215] -> w205
              frame Default {
              }
              frame 0.. {
                n84 = Get Drag Drop Data(8:"" ("type"), 9:w219) -> (3:w216:string)  [unwired: 1 in, 1 out]
                n85 = call "TrimShortcutPrefix.vi"("String in"=w216) -> ("String out"=w215:string)  [unwired: 18 in]
              }
            }
            n86 = case shown="True" w206 {
              tunnel: w205 -> [_ w214]
              tunnel: w204 -> [_ w213]
              frame False {
              }
              frame True {
                n87 = call "ChangeAssignedShortcut.vi"("QDKS Info"=w213, "Key"="", "QD"=w214) -> ()  [unwired: 8 in, 1 out]
              }
            }
            n88 = event-data("Accepted?"=w206) -> ()  [unwired: 1 in, 1 out]
          }
          event "1", "2", "3", "4", "5", "6", "7", "8", "9", "0", "Q", "W", "E", "R", "T", "A", "S", "D", "F", "G", "Z", "X", "C", "V", "B", "Y", "U", "I", "O", "P", "H", "J", "K", "L", "N", "M", "Shift": Drag Enter {
            n89 = event-data() -> ("Available Data Names"=w227:string[])  [unwired: 1 in]
            n90 = Search 1D Array(1D array=w227, element=w226) -> (index of element=w225:i32)  [unwired: 1 in]
            n91 = Greater Or Equal To 0?(x=w225) -> (x >= 0?=w224:bool)
            n92 = event-data("Accepted?"=w224) -> ()  [unwired: 1 in, 1 out]
          }
          event "1", "2", "3", "4", "5", "6", "7", "8", "9", "0", "Q", "W", "E", "R", "T", "A", "S", "D", "F", "G", "Z", "X", "C", "V", "B", "Y", "U", "I", "O", "P", "H", "J", "K", "L", "N", "M": Drop {
            # "/* Force Refresh */"
            n93 = event-data() -> ("CtlRef"=w236:refnum<vi>, "Available Data Names"=w239:string[])  [unwired: 1 in, 4 out]
            n94 = Search 1D Array(1D array=w239, element=w238) -> (index of element=w237:i32)  [unwired: 1 in]
            n95 = case shown="0.." w237 {
              tunnel: w238 -> [_ w250]
              tunnel: [_ TRUE] -> w235
              tunnel: w236 -> [_ w245]
              tunnel: [_ w246] -> w233
              tunnel: [_ w244] -> w234
              frame Default {
              }
              frame 0.. {
                n96 = property class="Bool"(reference=w245) -> ("Label.Text"=w244:string)  [unwired: 1 in, 2 out]
                n97 = Get Drag Drop Data(8:"" ("type"), 9:w250) -> (3:w247:string)  [unwired: 1 in, 1 out]
                n98 = call "TrimShortcutPrefix.vi"("String in"=w247) -> ("String out"=w246:string)  [unwired: 18 in]
              }
            }
            n99 = case shown="True" w235 {
              tunnel: w234 -> [_ w242]
              tunnel: w233 -> [_ w243]
              tunnel: w232 -> [_ w241]
              frame False {
              }
              frame True {
                n100 = call "ChangeAssignedShortcut.vi"("QDKS Info"=w241, "Key"=w242, "QD"=w243) -> ()  [unwired: 8 in, 1 out]
              }
            }
            n101 = event-data("Accepted?"=w235) -> ()  [unwired: 1 in, 1 out]
          }
          event "[Trigger]Refresh Btns": Value Change {
            n102 = event-data() -> ()  [unwired: 1 in, 4 out]
            n103 = property class="VI"() -> (error out=w259:errorcluster, "Panel"=w258:refnum<vi>)  [unwired: 2 in, 1 out]
            n104 = property class="Pnl"(reference=w258, error in=w259, "DeferPanUpdts"=TRUE ("Defer Panel Updates")) -> (reference out=w257:refnum<vi>, error out=w256:errorcluster)
            n105 = property class="Pnl"(reference=w257, error in=w256) -> (reference out=w268:refnum<vi>, error out=w270:errorcluster, "AllObjs[]"=w269:refnum<vi>[])
            n106 = call "FilterBooleanRefs.vi"("error in (no error)"=w270, "AllObjs[]"=w269) -> ("error out"=w265:errorcluster, "AllObjs[] (dup)"=w266:refnum<vi>[])  [unwired: 8 in]
            n107 = disable-structure shown="Enabled" {
              disable-tunnel: w266 -> [w277 _]
              disable-tunnel: w254 -> [w276 _]
              disable-tunnel: w265 -> [w275 w278]
              disable-tunnel: [w274 w278] -> w263
              disable-tunnel: [w273 _] -> w264
              disable-tunnel: w252 -> [w272 _]
              frame Enabled {
                n108 = call "PopulateToBooleanRef.vi"("CounterMap"=w272, "QDKS Info"=w276, "error in (no error)"=w275, "AllObjs[]"=w277) -> ("error out"=w274:errorcluster, "AllObjs[] (dup)"=w273:refnum<vi>[])  [unwired: 6 in]
              }
              frame Disabled {
              }
            }
            n109 = call "UpdateBooleanRef.vi"("error in (no error)"=w263, "AllObjs[]"=w264) -> ("error out"=w262:errorcluster)  [unwired: 8 in, 1 out]
            n110 = Close Reference(reference=w269, error in (no error)=w262) -> (error out=w267:errorcluster)
            n111 = Close Reference(reference=w268, error in (no error)=w267) -> (error out=w261:errorcluster)
            n112 = property class="Pnl"(reference=w258, error in=w261, "DeferPanUpdts"=FALSE ("Defer Panel Updates")) -> ()  [unwired: 2 out]
          }
          event "[Trigger]Update QSDK Info": Value Change {
            n113 = event-data() -> ()  [unwired: 1 in, 6 out]
            n114 = call <resource>:"QuickDrop Get QDKS Info for Shortcut Dialog.vi"() -> ("QDKS Info"=w283:T2[])  [unwired: 11 in]
            n115 = for {
              tunnel: w283 -> [w327] mode=indexing
              tunnel: [w326] -> w293 mode=indexing
              n116 = Unbundle By Name(w327) -> ("VI Name"=w326:string)
            }
            n117 = for {
              tunnel: w293 -> [w299] mode=indexing
              shift-right: [w298] -> w284
              shift-left: string[] [] -> [w297]
              shift-right: [w295] -> w281
              shift-left: i32[] [] -> [w294]
              i -> [w296]
              n118 = Search 1D Array(1D array=w297, element=w299) -> (index of element=w300:i32)  [unwired: 1 in]
              n119 = case shown="Default" w300 {
                tunnel: w299 -> [_ w308]
                tunnel: [w304 w306] -> w298
                tunnel: w297 -> [w304 w307]
                tunnel: w296 -> [w301 _]
                tunnel: [w302 w305] -> w295
                tunnel: w294 -> [w303 w305]
                frame Default {
                  n120 = Build Array (concatenate)(w303, w301) -> (w302:i32[])
                }
                frame -1 {
                  n121 = Build Array (concatenate)(w307, w308) -> (w306:string[])
                }
              }
            }
            n122 = for {
              tunnel: w283 -> [w313] mode=indexing
              tunnel: [w313] -> w282 mode=indexing if=w309
              tunnel: w281 -> [w312]
              i -> [w311]
              n123 = Search 1D Array(1D array=w312, element=w311) -> (index of element=w310:i32)  [unwired: 1 in]
              n124 = Less Than 0?(x=w310) -> (x < 0?=w309:bool)
            }
            n125 = call <resource>:"LV Config Read String.vi"("default value"="", "key"="QuickDrop_NEVSTOP_LAST_EXECUTE") -> ("value"=w291:string)  [unwired: 3 in, 2 out]
            n126 = call-poly <vilib>:"Trim Whitespace.vi"("string"=w291) -> ("trimmed string"=w292:string)  [unwired: 1 in]
            n127 = call "LoadCounterCfg.vi"() -> ("Variant"=w286:variant)  [unwired: 11 in]
            "Variant" <- w286
            n128 = case shown="Default" w292 {
              selector: w292 -> [w323 _]
              tunnel: [w318 w324] -> w287
              tunnel: w282 -> [w322 w325]
              tunnel: [w315 w325] -> w288
              tunnel: w284 -> [w314 w324]
              frame Default {
                n129 = Search 1D Array(1D array=w314, element=w323) -> (index of element=w321:i32)  [unwired: 1 in]
                n130 = Delete From Array(array=w322, index=w321) -> (deleted portion=w316:T2, array with subset deleted=w317:T2[])  [unwired: 1 in]
                n131 = Delete From Array(array=w314, index=w321) -> (deleted portion=w320:string, array with subset deleted=w319:string[])  [unwired: 1 in]
                n132 = Build Array (concatenate)(w316, w317) -> (w315:T2[])
                n133 = Build Array (concatenate)(w320, w319) -> (w318:string[])
              }
              frame "" {
              }
            }
          }
          event "Listbox": Mouse Down {
            n134 = event-data() -> ("CtlRef"=w330:refnum<vi>)  [unwired: 1 in]
            n135 = property class="LstBox (strict)"(reference=w330, "Key Focus"=FALSE) -> ()  [unwired: 1 in, 2 out]
          }
          event "[Trigger]Decorate List": Value Change {
            n136 = event-data() -> ()  [unwired: 1 in, 6 out]
            n137 = for {
              tunnel: w338 -> [w350] mode=indexing
              tunnel: [w343] -> w339 mode=indexing
              shift-right: [w344] -> w335
              shift-left: w336 -> [w347]
              n138 = Unbundle By Name(w350) -> ("VI Name"=w346:string, "Assigned Shortcut"=w349:string)
              n139 = Get Variant Attribute(Variant=w347, name=w346, default value (empty Variant)=0) -> (duplicate Variant=w344:variant, found=w341:bool, value=w342:i32)  [unwired: 1 in, 1 out]
              n140 = case shown="Default" w349 {
                selector: w349 -> [_ w358]
                tunnel: [_ w357] -> w348
                frame "" {
                }
                frame Default {
                  n141 = To Upper Case(1:w358) -> (0:w354:string)
                  n142 = Concatenate Strings("[" ("string"), w354, "] " ("string")) -> (w357:string)
                }
              }
              n143 = case shown="True" w341 {
                tunnel: w342 -> [_ w353]
                tunnel: [_ w351] -> w340
                frame False {
                }
                frame True {
                  n144 = Format Into String(format string="<%d> ", w353) -> (resulting string=w351:string)  [unwired: 2 in, 1 out]
                }
              }
              n145 = Concatenate Strings(w348, w340, w346) -> (w343:string)
            }
          }
        }
        n146 = case shown="False" w28 {
          tunnel: [w36 w39] -> w27
          tunnel: w26 -> [w37 w40]
          tunnel: w17 -> [_ w38]
          frame False {
            n147 = call "TrimShortcutPrefix.vi"("String in"=w37) -> ("String out"=w36:string)  [unwired: 18 in]
          }
          frame True {
            n148 = call "LookupQuickDrop.vi"("QDKS Info"=w38, "Key"=w40) -> ("QuickDrop"=w39:string)  [unwired: 8 in, 1 out]
          }
        }
        n149 = Not(x="Debug") -> (.not. x?=w29:bool)
        n150 = And(x=w29, y=w35) -> (x .and. y?=w31:bool)
      }
      n151 = call-poly <vilib>:"Trim Whitespace.vi"("string"=w12) -> ("trimmed string"=w9:string)  [unwired: 1 in]
      n152 = case shown="False" w7 {
        tunnel: w9 -> [w15 _]
        tunnel: w8 -> [w14 _]
        frame False {
          n153 = call "UpdateCounterCfg.vi"("name"=w15, "Variant"=w14) -> ()  [unwired: 10 in]
        }
        frame True {
        }
      }
    }
    frame Error {
    }
  }
  "Cancelled?" <- w6
  "error out" <- w4
  "QuckDrop" <- w3
  "Shift Pressed" <- w2
  "QDKS Info" <- w1
  n154 = disable-structure shown="Disabled" {
    frame Disabled {
      n155 = property on="[Trigger]Refresh Btns" class="Bool (strict)"("Val(Sgnl)"=TRUE ("Value (Signaling)")) -> ()  [unwired: 2 in, 2 out]
      n156 = property on="[Trigger]Update QSDK Info" class="Bool (strict)"("Val(Sgnl)"=TRUE ("Value (Signaling)")) -> ()  [unwired: 2 in, 2 out]
      n157 = property on="Listbox" class="LstBox (strict)" props=["Val(Sgnl)"]() -> ()  [unwired: 3 in, 2 out]
      n158 = local read "Listbox"() -> ()  [unwired: 1 out]
      n159 = property on="Listbox" class="LstBox (strict)"("Top Row"=0) -> ()  [unwired: 2 in, 2 out]
    }
    frame Enabled {
    }
  }
